vi "data_grid_v128_create_basemap.vi"(8 "Y_spacing":dbl format="%#_13g", 9 "X_spacing":dbl format="%#_13g", 10 "No. Rows":i32=16, 11 "No. Columns":i32=8) -> (2 "Grids_Unbounded":cluster{dbl[][], dbl[][], dbl[][]}, 3 "Grids_Bounded":cluster{dbl[][], dbl[][], dbl[][]})   [LabVIEW 2018]
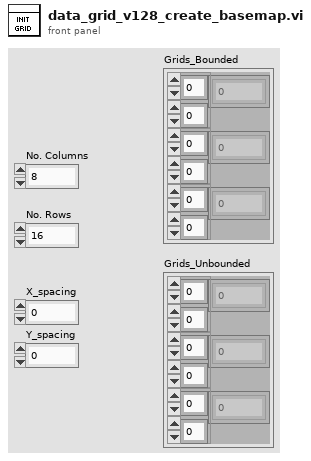
[diagram p1: front panel]
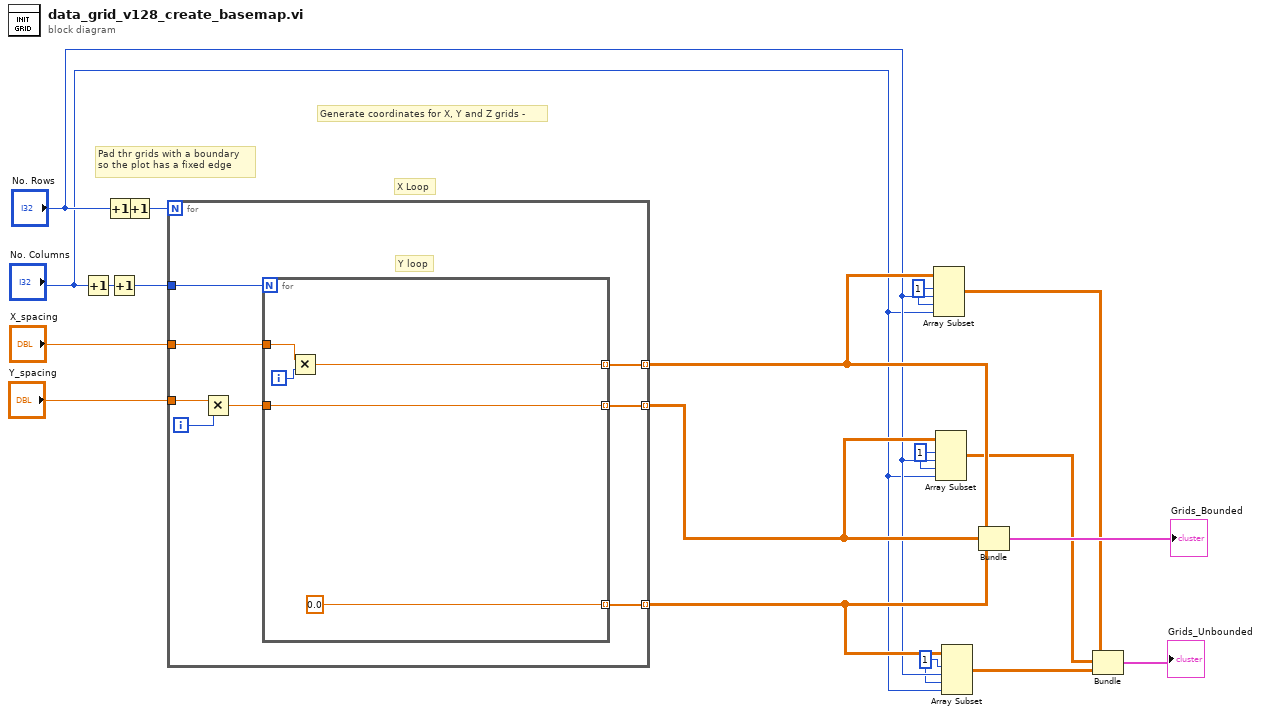
[diagram p0: block diagram]
diagram:
  w5 = 1 ("index")
  w9 = 1 ("index")
  w11 = 1 ("index")
  # "Pad thr grids with a boundary\nso the plot has a fixed edge"
  # "Generate coordinates for X, Y and Z grids -"
  # "X Loop"
  n1 = Increment(x="No. Columns") -> (x+1=w17:i32)
  n2 = Increment(x="No. Rows") -> (x+1=w19:i32)
  n3 = Increment(x=w17) -> (x+1=w16:i32)
  n4 = Increment(x=w19) -> (x+1=w18:i32)
  n5 = for {
    N: w18 -> [_]
    tunnel: [w27] -> w8 mode=indexing
    tunnel: w16 -> [w26]
    tunnel: "X_spacing" -> [w25]
    tunnel: "Y_spacing" -> [w23]
    tunnel: [w21] -> w12 mode=indexing
    tunnel: [w20] -> w10 mode=indexing
    i -> [w24]
    # "Y loop"
    n6 = Multiply(x=w23, y=w24) -> (x*y=w22:dbl)
    n7 = for {
      N: w26 -> [_]
      tunnel: [0.0 ("element")] -> w27 mode=indexing
      tunnel: w25 -> [w31]
      tunnel: w22 -> [w28]
      tunnel: [w29] -> w21 mode=indexing
      tunnel: [w28] -> w20 mode=indexing
      i -> [w30]
      n8 = Multiply(x=w31, y=w30) -> (x*y=w29:dbl)
    }
  }
  n9 = Array Subset(array=w12, index (row)=w11, length (row)="No. Rows", index (col)=w11, length (col)="No. Columns") -> (w2:dbl[][])
  n10 = Array Subset(array=w10, index (row)=w9, length (row)="No. Rows", index (col)=w9, length (col)="No. Columns") -> (w1:dbl[][])
  n11 = Array Subset(array=w8, index (row)=w5, length (row)="No. Rows", index (col)=w5, length (col)="No. Columns") -> (w3:dbl[][])
  n12 = Bundle(w12, w10, w8) -> (→"Grids_Bounded":cluster{dbl[][], dbl[][], dbl[][]})  [unwired: 1 in]
  n13 = Bundle(w2, w1, w3) -> (→"Grids_Unbounded":cluster{dbl[][], dbl[][], dbl[][]})  [unwired: 1 in]
